vi "Compile Knock Sensor Freq Scale.vi"(8 "error in (no error)":errorcluster, 9 "max rpm":dbl, 10 "max freq":dbl, 11 "min freq":dbl) -> (0 "error out":errorcluster, 2 "fxp intercept (b)":fxp<+,10,-10>, 3 "fxp slope (m)":fxp<+,16,-3>)   [LabVIEW 2019, in "Engine Simulation Toolkit System Explorer.lvlib"]
uses:
  Engine Simulation Toolkit System Explorer.lvlib
  <vilib>/rvi/Analysis/host/Public/NI_FpgaMspHost.lvlib
  Shared/Engine Simulation Toolkit Shared.lvlib
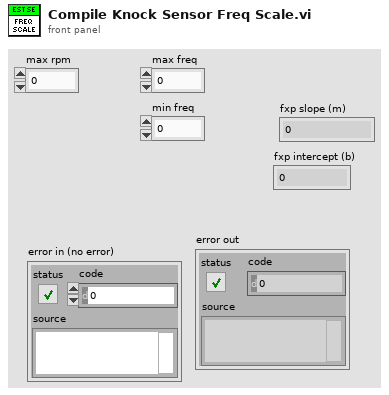
[diagram p1: front panel]
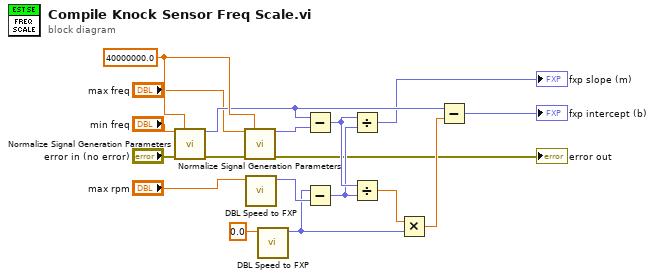
[diagram p0: block diagram]
diagram:
  w18 = 40000000.0 ("FPGA clock rate (Hz)")
  n1 = call <vilib>:"Normalize Signal Generation Parameters.vi"("frequency (Hz)"="min freq", "FPGA clock rate (Hz)"=w18, "error in (no error)"="error in (no error)") -> ("frequency (periods/tick)"=w10:fxp<+,32,0>, "error out"=w3:errorcluster)  [unwired: 7 in, 4 out]
  n2 = call <vilib>:"Normalize Signal Generation Parameters.vi"("frequency (Hz)"="max freq", "FPGA clock rate (Hz)"=w18, "error in (no error)"=w3) -> ("frequency (periods/tick)"=w17:fxp<+,32,0>, "error out"=→"error out":errorcluster)  [unwired: 7 in, 4 out]
  n3 = call "DBL Speed to FXP.vi"("Desired speed (RPM)"="max rpm") -> ("FXP speed"=w16:fxp<+/-,23,2>)  [unwired: 6 in, 4 out]
  n4 = call "DBL Speed to FXP.vi"("Desired speed (RPM)"=0.0 ("min rpm")) -> ("FXP speed"=w14:fxp<+/-,23,2>)  [unwired: 6 in, 4 out]
  n5 = Subtract(x=w10, y=w17) -> (x-y=w13:fxp<+/-,33,1>)
  n6 = Subtract(x=w14, y=w16) -> (x-y=w12:fxp<+/-,24,3>)
  n7 = Divide(x=w13, y=w12) -> (x/y=→"fxp slope (m)":fxp<+,16,-3>)
  n8 = Divide(x=w13, y=w12) -> (x/y=w11:dbl)
  n9 = Multiply(x=w11, y=w14) -> (x*y=w9:dbl)
  n10 = Subtract(x=w10, y=w9) -> (x-y=→"fxp intercept (b)":fxp<+,10,-10>)
